vi "Add_version_to_ERD.vi"(0 "session in":refnum<k35>, 1 "# of Iterations":i32, 5 "dst":i64, 9 "Read ERD":i64[](array[numeric]) format="%x", 11 "error in":errorcluster) -> (8 "ERD_Data_Out":T1[](array[typedef]) {"ERD Number" format="%x"}, 15 "error out":errorcluster)   [LabVIEW 2021]
uses:
  Controles/Read_ERD.ctl
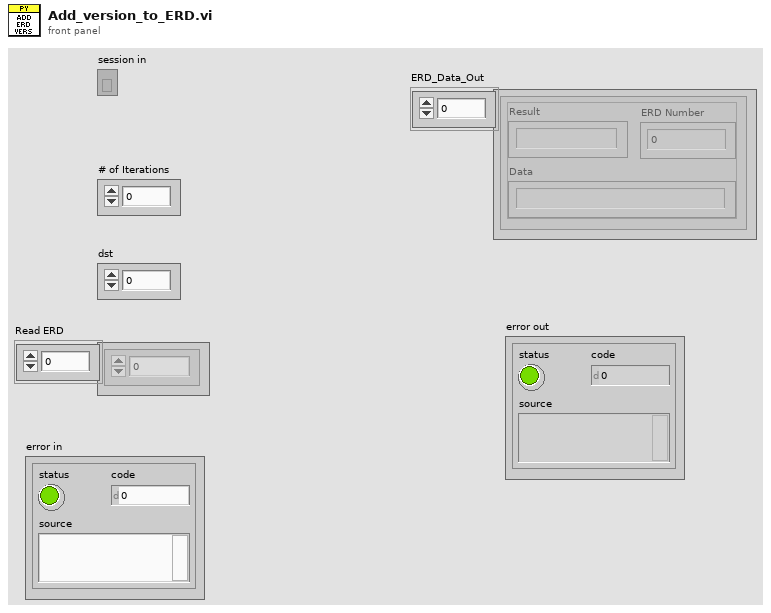
[diagram p1: front panel]
types:
  T1 = typedef "Read_ERD.ctl" = cluster{"Result":string, "ERD Number":i64, "Data":string}
  T2 = typedef "Multiple_Read_ERD.ctl" = T1[]
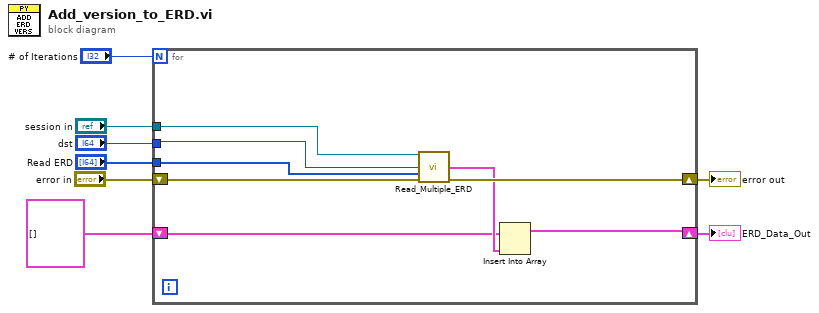
[diagram p0: block diagram]
diagram:
  n1 = for {
    N: "# of Iterations" -> [_]
    tunnel: "session in" -> [w16]
    tunnel: "dst" -> [w15]
    tunnel: "Read ERD" -> [w14]
    shift-right: [w12] -> w1
    shift-left: "error in" -> [w13]
    shift-right: [w9] -> w2
    shift-left: T1[] [] ("array") -> [w10]
    n2 = call "Read_Multiple_ERD.vi"("session in"=w16, "dst"=w15, "Read ERD"=w14, "error out"=w13) -> ("Multiple Read"=w11:T2, "error IO"=w12:errorcluster)  [unwired: 9 in, 1 out]
    n3 = Insert Into Array(array=w10, new element=w11) -> (w9:T1[])  [unwired: 1 in]
  }
  "ERD_Data_Out" <- w2
  "error out" <- w1
